vi "Test Seeleccion servicio Taxi.vi"(8 "error in (no error)":errorcluster, 11 "TestCase in":refnum<class "Unit Test Proy.lvclass">) -> (0 "error out":errorcluster, 3 "TestCase out":refnum<class "Unit Test Proy.lvclass">)   [LabVIEW 2020, in "Unit Test Proy.lvclass"]
uses:
  Unit Test Proy.lvclass
  Paquetes/Paquetes.lvclass
  Paquetes/Paquetes.lvclass/Paquetes.ctl
  Unit Test Proy.lvclass/Unit Test Proy.ctl
  <vilib>/addons/_JKI Toolkits/VI Tester/TestCase.llb/TestCase.lvclass
  C:/Program Files (x86)/National Instruments/LabVIEW 2020/vi.lib/addons/_JKI Toolkits/VI Tester/TestCase.llb/TestCase.lvclass
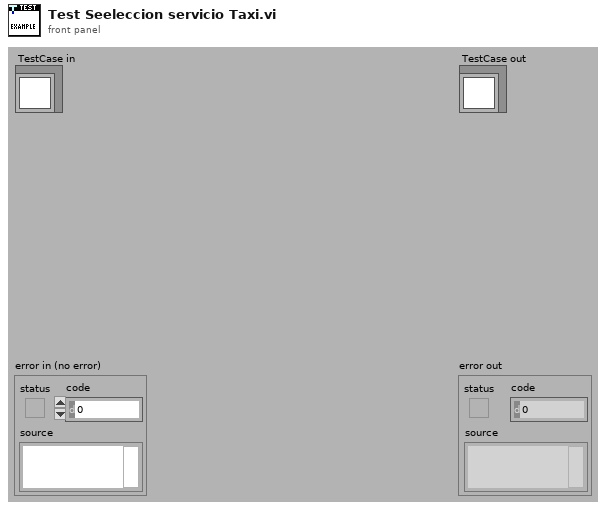
[diagram p1: front panel]
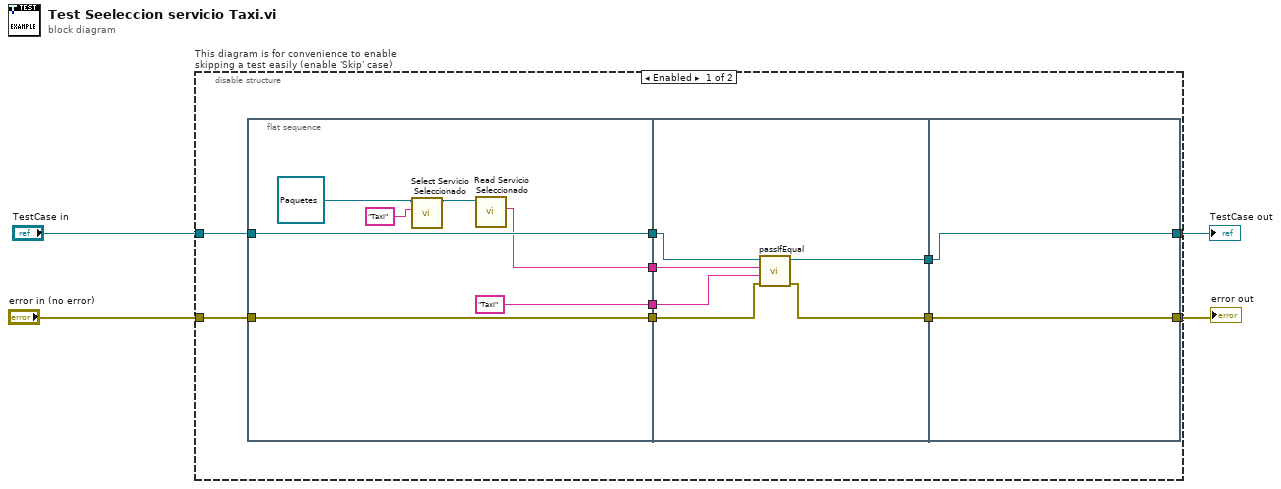
[diagram p0: block diagram]
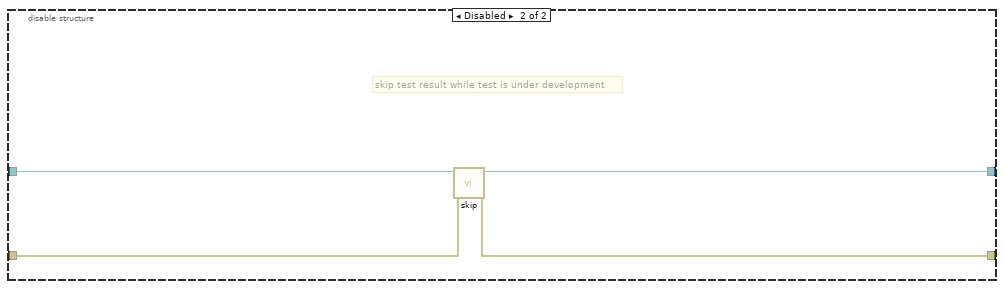
[diagram p2: hidden frame]
diagram:
  n1 = disable-structure "This diagram is for convenience to enable skipping a test easily (enable 'Skip' case)" shown="Enabled" {
    disable-tunnel: "TestCase in" -> [w14 w33]
    disable-tunnel: [w10 w31] -> w1
    disable-tunnel: [w9 w32] -> w3
    disable-tunnel: "error in (no error)" -> [w13 w30]
    frame Enabled {
      n2 = flat-sequence {
        tunnel: w14 -> [w21]
        tunnel: w13 -> [w20]
        tunnel: [w21] -> w12
        tunnel: [w20] -> w7
        tunnel: [w19] -> w6
        tunnel: ["Taxi"] -> w5
        tunnel: w12 -> [w27]
        tunnel: [w26] -> w11
        tunnel: [w25] -> w8
        tunnel: w7 -> [w24]
        tunnel: w6 -> [w22]
        tunnel: w5 -> [w23]
        tunnel: w11 -> [w29]
        tunnel: [w29] -> w10
        tunnel: [w28] -> w9
        tunnel: w8 -> [w28]
        frame #0 {
          n3 = call "Select Servicio Seleccionado.vi"("Servicio Seleccionado"="Taxi" ("Servicio"), "Paquetes in"=refnum<class "Paquetes.lvclass"> refnum ("Paquetes.lvlib:Paquetes.lvclass")) -> ("Paquetes out"=w15:refnum<class "Paquetes.lvclass">)  [unwired: 8 in, 1 out]
          n4 = call "Read Servicio Seleccionado.vi"("Paquetes in"=w15) -> ("Servicio Seleccionado"=w19:string)  [unwired: 8 in, 2 out]
        }
        frame #1 {
          n5 = call-dynamic "passIfEqual.vi"("error in (no error)"=w24, "y"=w23, "x"=w22, "TestCase in"=w27) -> ("error out"=w25:errorcluster, "TestCase out"=w26:refnum<class "Unit Test Proy.lvclass">)  [unwired: 6 in]
        }
        frame #2 {
        }
      }
    }
    frame Disabled {
      # "skip test result while test is under development"
      n6 = call <vilib>:"skip.vi"("error in (no error)"=w30, "TestCase in"=w33) -> ("error out"=w32:errorcluster, "TestCase out"=w31:refnum<class "Unit Test Proy.lvclass">)  [unwired: 8 in]
    }
  }
  "error out" <- w3
  "TestCase out" <- w1
